vi "BuildCall.vi"(7 "PythonConverter_BD in":refnum<class "PyConvBD.lvclass">, 8 "error in":errorcluster, 11 "Diagram in":refnum<class "Diagram.lvclass">) -> (0 "error out":errorcluster, 3 "Diagram out":refnum<class "Diagram.lvclass">, 4 "diagram":string, 5 "PythonConverter_BD out":refnum<class "PyConvBD.lvclass">)   [LabVIEW 2014, in "Diagram.lvclass"]
uses:
  Diagram.lvclass
  Python/PythonConverter_BD/PyConvBD.lvclass
  Python/Parsing/ClassTypeTD.ctl
  CollectTD.ctl
  Diagram.lvclass/Diagram.ctl
  VI_AST/VI_AST.lvclass/VI_AST.ctl
  Python/Parsing/Python Functions.lvlib
  VI_AST/VI_AST.lvclass
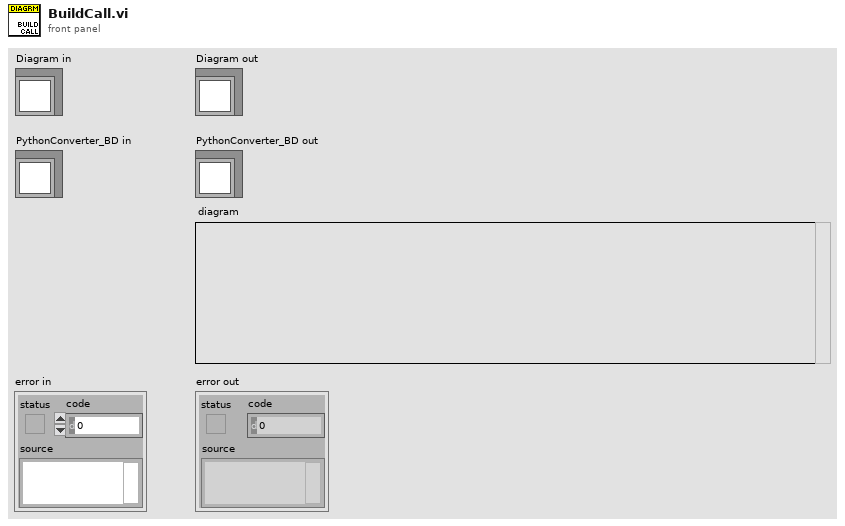
[diagram p1: front panel]
types:
  T1 = typedef "CollectTD.ctl" = cluster{"Rank":i32, "collect":string, "branches":string[]}
  T2 = typedef "Python Functions.lvlib/ClassTypeTD.ctl" = enum16{"class", "function"}
  T3 = typedef "NodeCall_TD.ctl" = cluster{"call":string, "collect":string, "Threaded":bool, "branches":string[]}
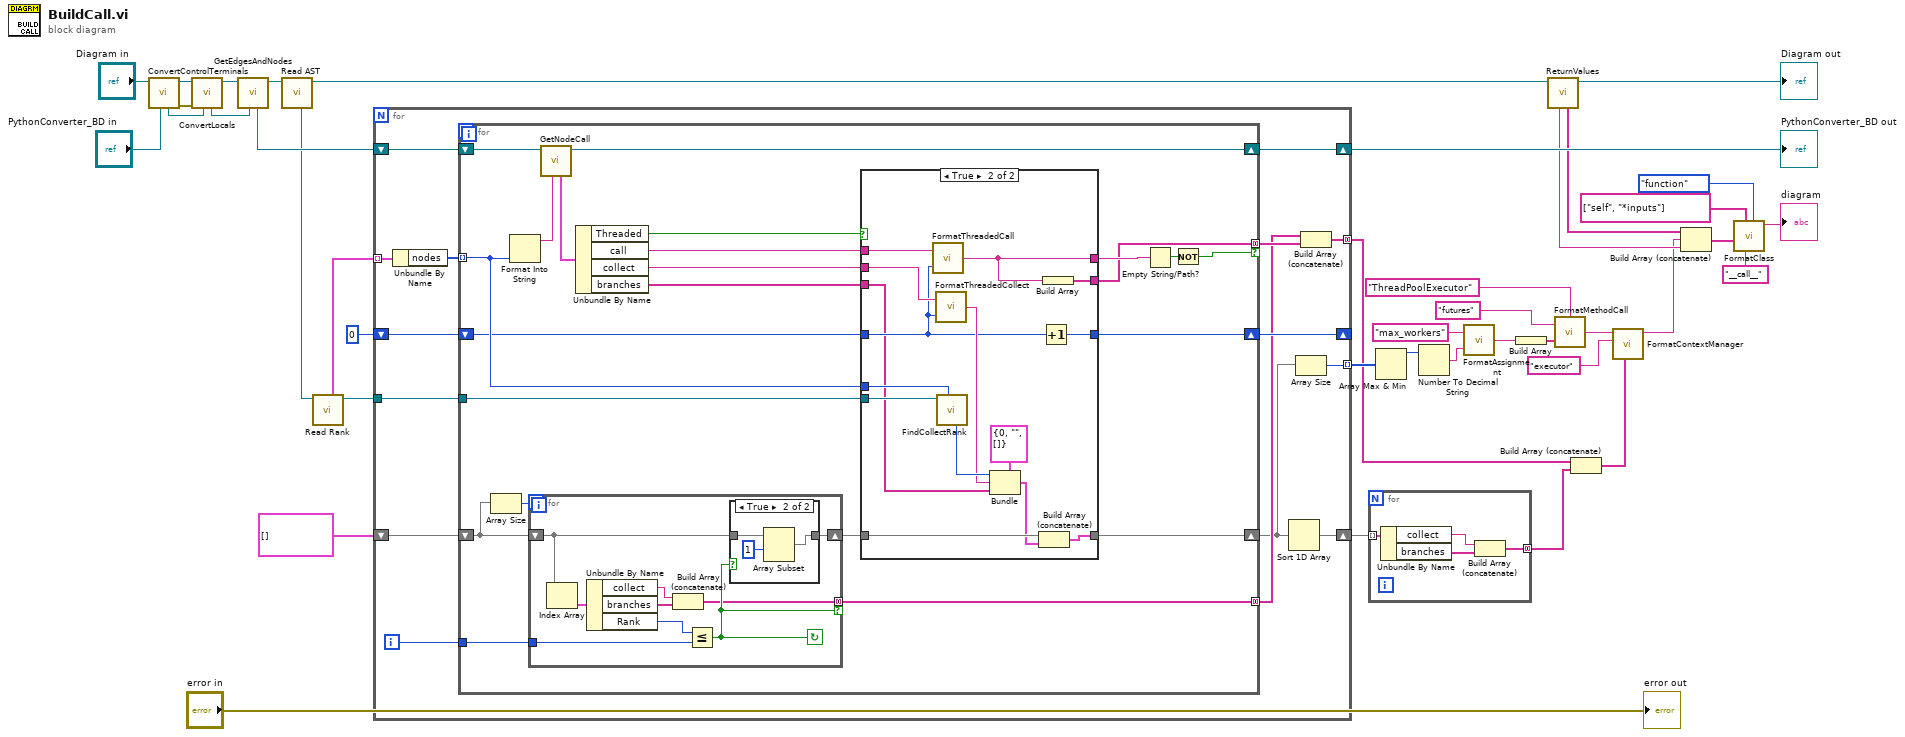
[diagram p0: block diagram]
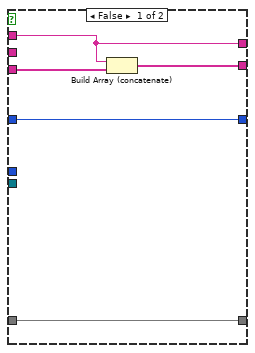
[diagram p3: hidden frame]
diagram:
  n1 = call "ConvertControlTerminals.vi"("PythonConverter_BD in"="PythonConverter_BD in", "Diagram in"="Diagram in") -> ("error out"=w4:errorcluster, "Diagram out"=w5:refnum<class "Diagram.lvclass">, "PythonConverter_BD out"=w2:refnum<class "PyConvBD.lvclass">)  [unwired: 5 in]
  n2 = call "ConvertLocals.vi"("PythonConverter_BD in"=w2, "error in"=w4, "Diagram in"=w5) -> ("Diagram out"=w3:refnum<class "Diagram.lvclass">, "PythonConverter_BD out"=w1:refnum<class "PyConvBD.lvclass">)  [unwired: 4 in, 1 out]
  n3 = call "GetEdgesAndNodes.vi"("PythonConverter_BD in"=w1, "Diagram in"=w3) -> ("Diagram out"=w28:refnum<class "Diagram.lvclass">, "PythonConverter_BD out"=w29:refnum<class "PyConvBD.lvclass">)  [unwired: 6 in]
  n4 = call "Read AST.vi"("Diagram in"=w28) -> ("Diagram out"=w27:refnum<class "Diagram.lvclass">, "AST"=w26:refnum<class "VI_AST.lvclass">)  [unwired: 7 in]
  n5 = call "Read Rank.vi"("VI_AST in"=w26) -> ("VI_AST out"=w24:refnum<class "VI_AST.lvclass">, "Rank"=w25:cluster{"nodes":i32[]}[])  [unwired: 7 in]
  n6 = for {
    tunnel: w25 -> [w55] mode=indexing
    shift-right: [w52] -> w40
    shift-left: w29 -> [w53]
    tunnel: [w50] -> w8 mode=concatenating
    tunnel: w24 -> [w49]
    shift-right: [w47] -> w21
    shift-left: T1[] [] -> [w48]
    shift-right: [w44] -> _
    shift-left: 0 -> [w45]
    tunnel: [w42] -> w19 mode=indexing
    i -> [w46]
    n7 = Unbundle By Name(w55) -> ("nodes"=w54:i32[])
    n8 = for {
      tunnel: w54 -> [w67] mode=indexing
      shift-right: [w76] -> w52
      shift-left: w53 -> [w77]
      tunnel: [w56] -> w51 mode=concatenating if=w73
      tunnel: w49 -> [w66]
      shift-right: [w64] -> w41
      shift-left: w48 -> [w59]
      tunnel: w46 -> [w68]
      tunnel: [w63] -> w43 mode=concatenating
      shift-right: [w61] -> w44
      shift-left: w45 -> [w62]
      n9 = Array Size(array=w59) -> (size(s)=w60:i32)
      n10 = Format Into String(w67) -> (resulting string=w75:string)  [unwired: 3 in, 1 out]
      n11 = for {
        N: w60 -> [_]
        shift-right: [w83] -> w65
        shift-left: w59 -> [w84]
        tunnel: w68 -> [w85]
        tunnel: [w78] -> w63 mode=concatenating if=w82
        stop <- w82 continue-if-true
        n12 = Index Array(array=w84) -> (element=w86:T1)  [unwired: 1 in]
        n13 = Unbundle By Name(w86) -> ("collect"=w80:string, "branches"=w79:string[], "Rank"=w81:i32)
        n14 = Build Array (concatenate)(w80, w79) -> (w78:string[])
        n15 = Less Or Equal?(x=w81, y=w85) -> (x <= y?=w82:bool)
        n16 = case shown="True" w82 {
          tunnel: w84 -> [w87 w90]
          tunnel: [w87 w89] -> w83
          frame False {
          }
          frame True {
            n17 = Array Subset(array=w90, index=1) -> (w89:T1[])  [unwired: 1 in]
          }
        }
      }
      n18 = call "GetNodeCall.vi"("name"=w75, "PythonConverter_BD in"=w77) -> ("PythonConverter_BD out"=w76:refnum<class "PyConvBD.lvclass">, "call"=w72:T3)  [unwired: 5 in, 1 out]
      n19 = Unbundle By Name(w72) -> ("Threaded"=w71:bool, "call"=w70:string, "collect"=w69:string, "branches"=w58:string[])
      n20 = case shown="True" w71 {
        tunnel: [w92 w97] -> w57
        tunnel: w70 -> [w92 w110]
        tunnel: w69 -> [_ w109]
        tunnel: w62 -> [w94 w101]
        tunnel: w67 -> [_ w108]
        tunnel: w66 -> [_ w107]
        tunnel: w65 -> [w95 w104]
        tunnel: [w95 w102] -> w64
        tunnel: [w94 w100] -> w61
        tunnel: w58 -> [w93 w98]
        tunnel: [w91 w96] -> w56
        frame False {
          n21 = Build Array (concatenate)(w92, w93) -> (w91:string[])
        }
        frame True {
          n22 = call "FormatThreadedCall.vi"("thread #"=w101, "call"=w110) -> ("python object"=w97:string)  [unwired: 1 in]
          n23 = call "FormatThreadedCollect.vi"("thread #"=w101, "collect"=w109) -> ("python object"=w105:string)  [unwired: 1 in]
          n24 = call "FindCollectRank.vi"("UID"=w108, "VI_AST in"=w107) -> ("collect rank"=w106:i32)  [unwired: 6 in, 1 out]
          n25 = Bundle(cluster=T1 {"Rank"=0, "collect"="", "branches"=[]}, "Rank"=w106, "collect"=w105, "branches"=w98) -> (w103:T1)
          n26 = Build Array (concatenate)(w104, w103) -> (w102:T1[])
          n27 = Increment(x=w101) -> (x+1=w100:i32)
          n28 = Build Array(w97) -> (w96:string[])
        }
      }
      n29 = Empty String/Path?(string/path=w57) -> (empty?=w74:bool)
      n30 = Not(x=w74) -> (.not. x?=w73:bool)
    }
    n31 = Sort 1D Array(array=w41) -> (sorted array=w47:T1[])
    n32 = Array Size(array=w41) -> (size(s)=w42:i32)
    n33 = Build Array (concatenate)(w43, w51) -> (w50:string[])
  }
  "PythonConverter_BD out" <- w40
  n34 = for {
    tunnel: w21 -> [w114] mode=indexing
    tunnel: [w111] -> w7 mode=concatenating
    n35 = Unbundle By Name(w114) -> ("collect"=w113:string, "branches"=w112:string[])
    n36 = Build Array (concatenate)(w113, w112) -> (w111:string[])
  }
  n37 = Array Max & Min(array=w19) -> (max value=w18:i32)  [unwired: 3 out]
  n38 = Number To Decimal String(number=w18) -> (decimal integer string=w17:string)  [unwired: 1 in]
  n39 = call "FormatAssignment.vi"("value"=w17, "name"="max_workers") -> ("python assignment"=w15:string)
  n40 = Build Array(w15) -> (w14:string[])
  n41 = call-dynamic "ReturnValues.vi"("Diagram in"=w27) -> ("Diagram out"=→"Diagram out":refnum<class "Diagram.lvclass">, "inputs"=w31:string[], "return"=w20:string)  [unwired: 5 in, 1 out]
  n42 = call "FormatMethodCall.vi"("method"="ThreadPoolExecutor", "parameters"=w14, "object"="futures") -> ("python object"=w11:string)
  n43 = Build Array (concatenate)(w8, w7) -> (w6:string[])
  n44 = call "FormatContextManager.vi"("body"=w6, "name"="executor", "manager"=w11) -> ("python"=w9:string)  [unwired: 6 in]
  n45 = Build Array (concatenate)(w31, w9, w20) -> (w32:string[])
  n46 = call "FormatClass.vi"("type"=ClassTypeTD."function", "name"="__call__", "parameters/ancestors"=string[] ["self", "*inputs"], "body"=w32) -> ("python"=→"diagram":string)  [unwired: 7 in]
  "error out" <- "error in"
